vi "Main Game Controller.vi"(8 "error in (no error)":errorcluster, 11 "output cluster":refnum<class "Game.lvclass">) -> (0 "error out":errorcluster)   [LabVIEW 2021, in "Game.lvclass"]
uses:
  Application/Game.lvclass
  GameEl_class/private/Enum Direction.ctl
  Application/Shield.ctl
  Application/Grapes.ctl
  Application/Backgroud_v2.ctl
  <vilib>/Platform/TimedLoop/XDataNode/timing_clust.ctl
  <vilib>/Platform/TimedLoop/XDataNode/nitl_modes.ctl
  <vilib>/Platform/TimedLoop/XDataNode/wakeup.ctl
  Application/Game.lvclass/Game.ctl
  e26eec9f-965e-4c3b-b51e-9e299e1f8818.vi
  49b93924-5950-4f5a-b15f-497dbc55912f.vi
  Application/Globales Snake.vi
  <vilib>/platform/TimedLoop/XDataNode/XDataNode.xnode
  GameEl_class/GameEl.lvclass
  Snake_class/Snake.lvclass
  <vilib>/Platform/TimedLoop/XDataNode/XDNodeRunTimeDep.lvlib
  Board Game_class/Board Game.lvclass
  Imposible_Snake_v2/LVApp/Modules/Sound Manager/Sound Manager.lvlib
panel:
  out "Image Ring":u16(ring)
  out "Star":bool
  in  "Grapes":T1
  in  "Shield":T2
  in  "Studios":bool caption="Creator 2"
  in  "Creator":bool
  out "TIME":string
  out "SCORE":string
  out "Board Game":u32[][](array[colorbox])
  out "Background":T3=1
  in  "Usert Stop Game":bool
  in  "Pause/Resume":bool
  out "Direction":T4
  out "Current Score":u16
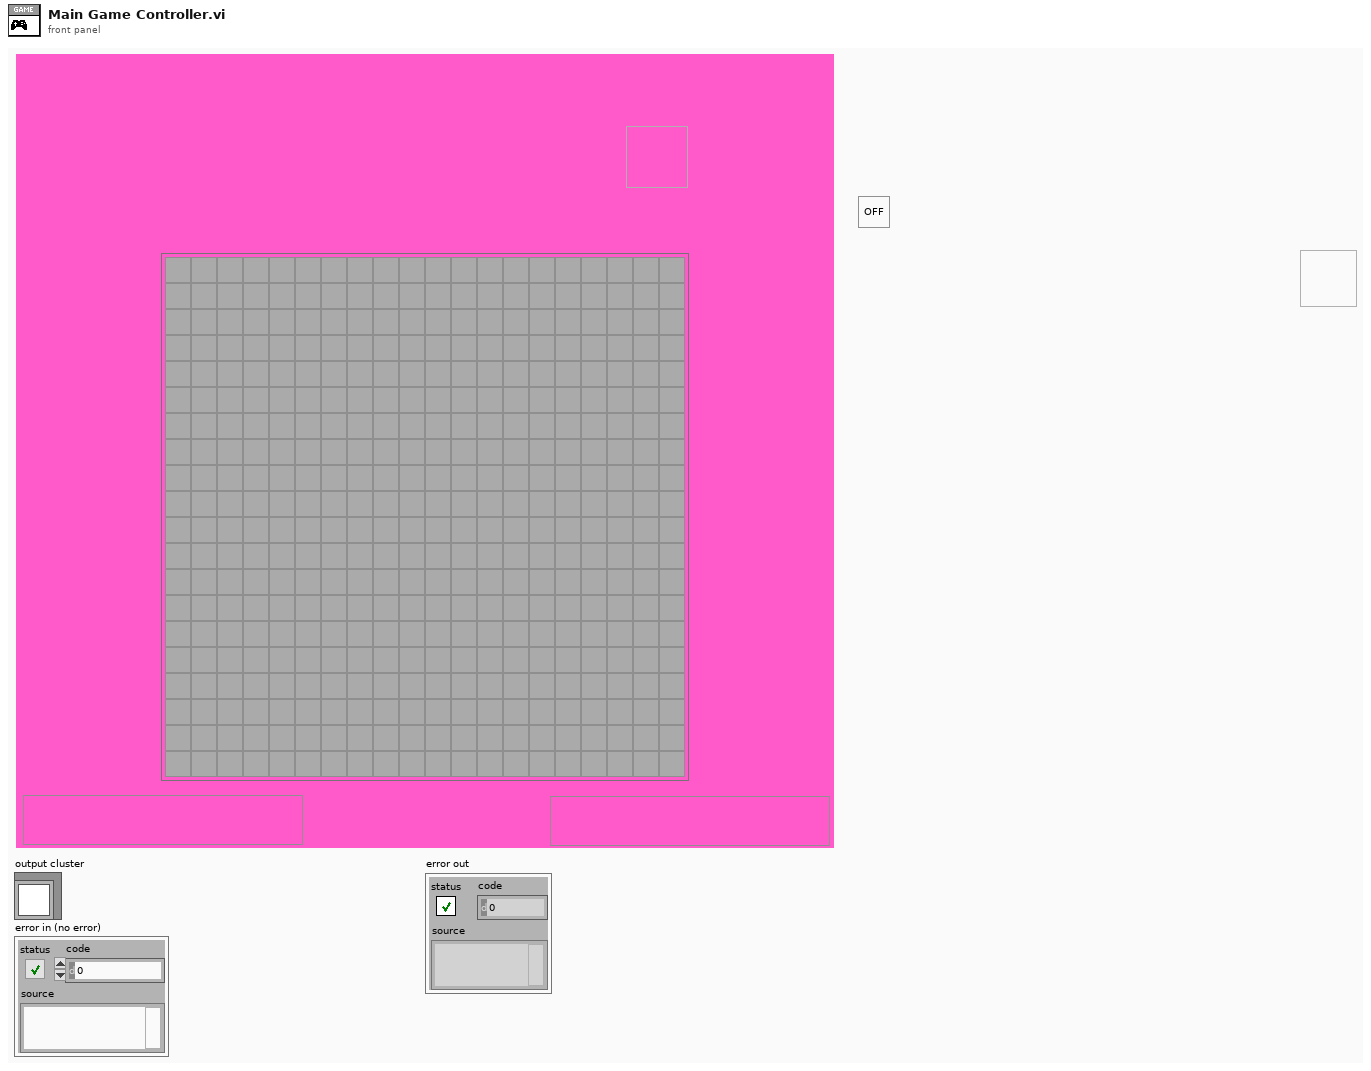
[diagram p1: front panel]
types:
  T1 = typedef "Game.lvclass/Grapes.ctl" = u16
  T2 = typedef "Game.lvclass/Shield.ctl" = u16
  T3 = typedef "Game.lvclass/Backgroud_v2.ctl" = u16
  T4 = typedef "GameEl.lvclass/Enum Direction.ctl" = enum16{"Up", "Down", "Forward", "Backward"}
  T5 = typedef "XDNodeRunTimeDep.lvlib/timing_clust.ctl" = cluster{"Expected End [f-1]":u64, "Actual End [f-1]":u64, "Finished Late? [f-1]":bool, "Expected End [i-1]":u64, "Actual End [i-1]":u64, "Finished Late? [i-1]":bool, "Expected Start [i]":u64, "Actual Start [i]":u64, "Expected Start [f]":u64, "Actual Start [f]":u64, "Source Name":string, "Structure Name":string, "Period":i64, "Deadline":i64, "Offset":i64, "Start":i64, "Priority":i32, "Timeout":i32, "Mode":T6, "Wakeup Reason":T7, "Error":errorcluster, "Source Type":string, "Secondary Source Type":string, "Global End Time":u64, "Global Start Time":u64, "Frame Duration":u64, "Iteration Duration":u64, "Assigned CPU":i32, "I/O Scan Engine Mode":u32}
  T6 = typedef "XDNodeRunTimeDep.lvlib/nitl_modes.ctl" = enum32{"No Change", "Process missed periods, maintain original phase", "Discard missed periods, maintain original phase", "Process missed periods, ignore original phase", "Discard missed periods, ignore original phase"}
  T7 = typedef "XDNodeRunTimeDep.lvlib/wakeup.ctl" = enum32{"Normal", "Aborted", "Asynchronous wakeup", "Timing source error", "Timed loop error", "Timeout"}
  T8 = enum8{"Enabled", "Disabled", "Disabled and Grayed Out"}
  T9 = cluster{"Event Registration Refnum":refnum<event-registration>}
  T10 = enum32{"invalid app kind", "Development System", "Run Time System", "Student Edition", "Embedded LabVIEW", "Evaluation", "Custom"}
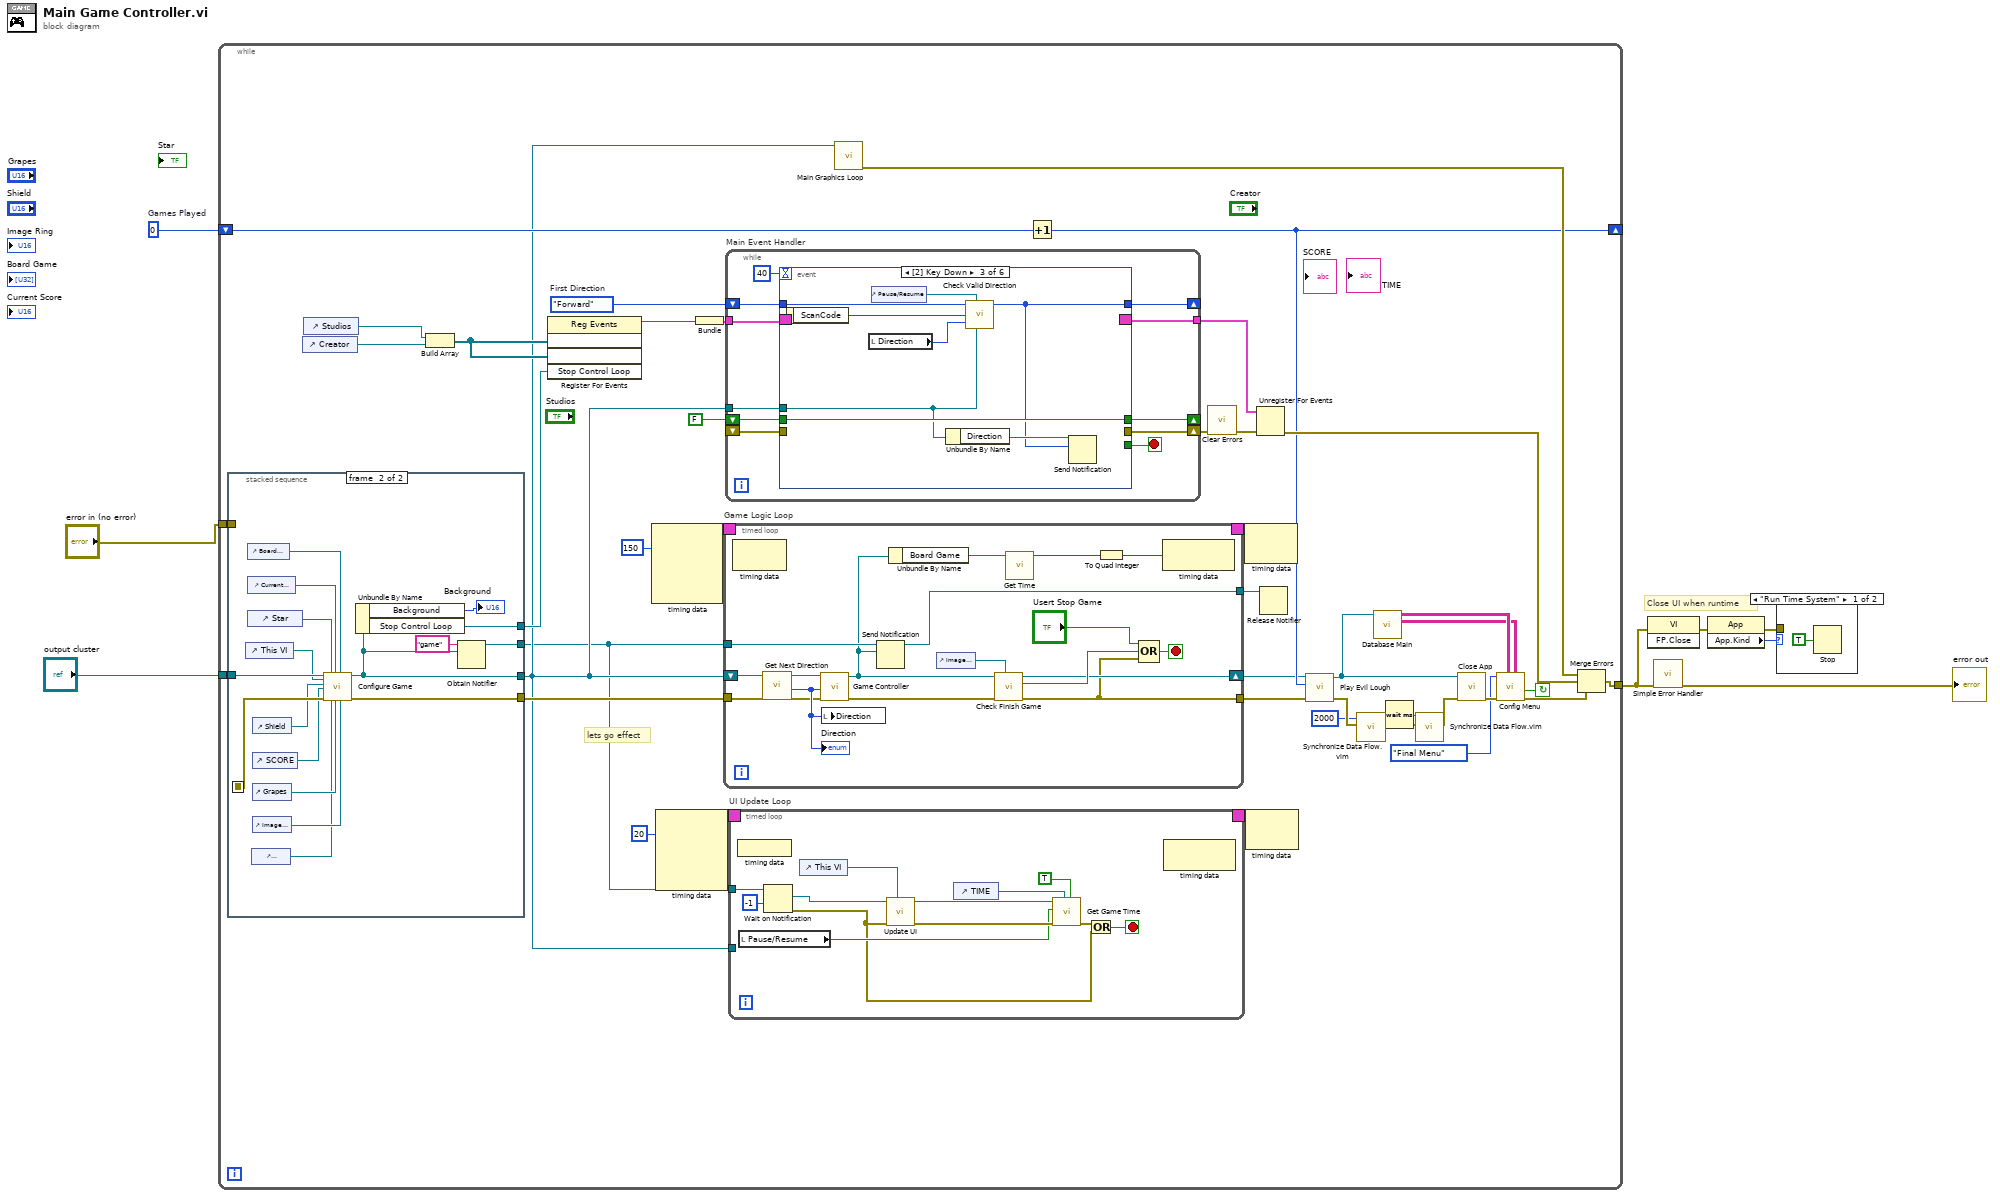
[diagram p0: block diagram]
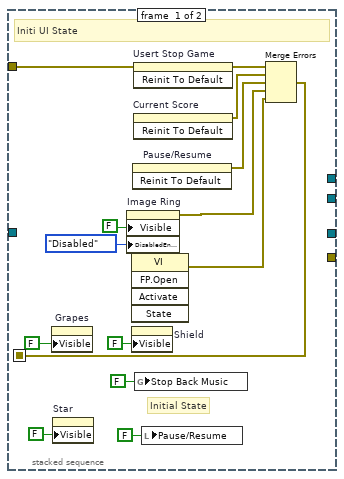
[diagram p2: hidden frame]
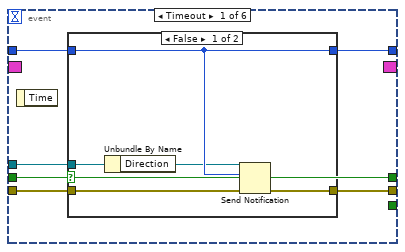
[diagram p3: hidden frame]
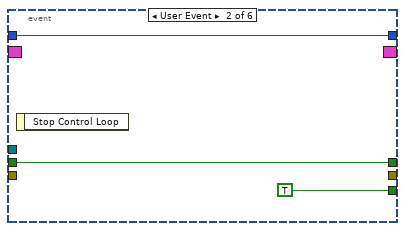
[diagram p5: hidden frame]
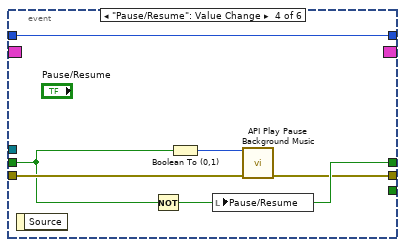
[diagram p6: hidden frame]
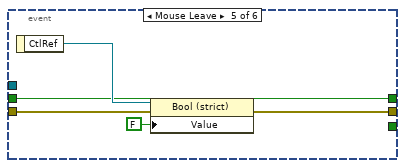
[diagram p7: hidden frame]
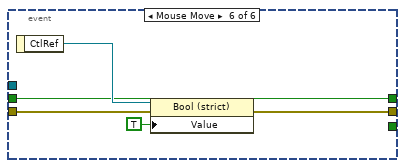
[diagram p8: hidden frame]
diagram:
  w8 = 0  # Games Played
  # "Close UI when runtime"
  n1 = while {
    tunnel: [w43] -> w5
    tunnel: "output cluster" -> [w41]
    shift-right: [w39] -> _
    shift-left: w8 -> [w40]
    tunnel: "error in (no error)" -> [w10]
    stop <- w34 continue-if-true
    w50 = Enum_Direction."Forward"  # First Direction
    # "lets go effect"
    n2 = stacked-sequence {
      seq-local: [w105 _] -> [_ w126]
      tunnel: [_ w125] -> w29
      tunnel: [_ w111] -> w13
      tunnel: [_ w122] -> w44
      tunnel: w41 -> [_ w117]
      tunnel: [_ w110] -> w12
      tunnel: w10 -> [w96 _]
      frame #0 {
        # "Initial State"
        # "Initi UI State"
        n3 = property on="Grapes" class="Ring (strict)"("Visible"=FALSE) -> ()  [unwired: 2 in, 2 out]
        n4 = property on="Star" class="Bool (strict)"("Visible"=FALSE) -> ()  [unwired: 2 in, 2 out]
        n5 = property on="Image Ring" class="Ring (strict)"("Visible"=FALSE, "DisabledEnum"=T8."Disabled" ("Disabled")) -> (error out=w101:errorcluster)  [unwired: 2 in, 1 out]
        n6 = invoke class="VI" method="FP.Open"() -> (error out=w106:errorcluster)  [unwired: 5 in, 4 out]
        n7 = property on="Shield" class="Ring (strict)"("Visible"=FALSE) -> ()  [unwired: 2 in, 2 out]
        n8 = invoke on="Pause/Resume" class="Bool (strict)" method="Reinit To Default"() -> (error out=w107:errorcluster)  [unwired: 3 in, 2 out]
        n9 = invoke on="Usert Stop Game" class="Bool (strict)" method="Reinit To Default"(error in=w96) -> (error out=w109:errorcluster)  [unwired: 2 in, 2 out]
        n10 = invoke on="Current Score" class="DigNum (strict)" method="Reinit To Default"() -> (error out=w108:errorcluster)  [unwired: 3 in, 2 out]
        n11 = global write "Globales Snake.vi" "Stop Back Music"(FALSE ("Stop Back Music")) -> ()
        n12 = local write "Pause/Resume"(FALSE ("Pause/Resume")) -> ()
        n13 = Merge Errors(w109, w108, w107, w101, w106) -> (w105:errorcluster)
      }
      frame #1 {
        n14 = control-ref of="This VI"() -> (w113:refnum<vi>)
        n15 = control-ref of="Board Game"() -> (w124:refnum<vi>)
        n16 = control-ref of="Current Score"() -> (w123:refnum<vi>)
        n17 = control-ref of="Star"() -> (w114:refnum<vi>)
        n18 = control-ref of="Background"() -> (w116:refnum<vi>)
        n19 = control-ref of="Shield"() -> (w121:refnum<vi>)
        n20 = control-ref of="SCORE"() -> (w120:refnum<vi>)
        n21 = control-ref of="Grapes"() -> (w119:refnum<vi>)
        n22 = control-ref of="Image Ring"() -> (w118:refnum<vi>)
        n23 = call "Configure Game.vi"("input cluster"=w117, "This VI"=w113, "Shield"=w121, "SCORE"=w120, "error in (no error)"=w126, "STAR"=w114, "Background"=w116, "Score"=w123, "Grapes"=w119, "Board Game"=w124, "Image Ring"=w118) -> ("Application out"=w111:refnum<class "Game.lvclass">, "error out"=w125:errorcluster)  [unwired: 7 in]
        n24 = Unbundle By Name(w111) -> ("Background"=→"Background":u16, "Stop Control Loop"=w122:refnum<user-event>)
        n25 = Obtain Notifier(name (unnamed)="game", notification data type=w111) -> (notifier out=w110:refnum<notifier>)  [unwired: 2 in, 2 out]
      }
    }
    n26 = control-ref of="Creator"() -> (w28:refnum<vi>)
    n27 = control-ref of="Studios"() -> (w27:refnum<vi>)
    n28 = Build Array(w27, w28) -> (w26:refnum<vi>[])
    n29 = register-events(w26, w26, w44) -> (reference out=w51:refnum<event-registration>)  [unwired: 2 in, 1 out]
    n30 = node-c288(i64 150 ("Period")) -> (w18:T5)  [unwired: 3 in]
    n31 = node-c288(i64 20 ("Period")) -> (w15:T5)  [unwired: 3 in]
    n32 = Bundle("Event Registration Refnum"=w51) -> (w30:T9)  [unwired: 1 in]
    n33 = timed-loop "Game Logic Loop" {
      tunnel: w29 -> [w81]
      tunnel: [w77] -> w37
      shift-right: [w79] -> w38
      shift-left: w13 -> [w86]
      timing: w18 -> [_]
      timing-out: [_] -> w17
      tunnel: w12 -> [w73]
      tunnel: [w70] -> w9
      stop <- w71 stop-if-true
      n34 = node-c288() -> ()  [unwired: 1 in, 1 out]
      n35 = call "Get Next Direction.vi"("error in (no error)"=w81, "Application in"=w86) -> ("error out"=w78:errorcluster, "Direction"=w83:T4, "Application out"=w85:refnum<class "Game.lvclass">)  [unwired: 7 in]
      "Direction" <- w83
      n36 = call "Game Controller.vi"("error in (no error)"=w78, "Direction"=w83, "Application in"=w85) -> ("error out"=w80:errorcluster, "Application out"=w72:refnum<class "Game.lvclass">)  [unwired: 7 in]
      n37 = local write "Direction"(w83) -> ()
      n38 = Send Notification(notification=w72, notifier=w73) -> (notifier out=w70:refnum<notifier>)  [unwired: 1 in, 1 out]
      n39 = Unbundle By Name(w72) -> ("Board Game"=w76:refnum<class "Board Game.lvclass">)
      n40 = control-ref of="Image Ring"() -> (w84:refnum<vi>)
      n41 = call "Check Finish Game.vi"("Game Result"=w84, "error in (no error)"=w80, "Application in"=w72) -> ("error out"=w77:errorcluster, "Finish Game?"=w82:bool, "Application out"=w79:refnum<class "Game.lvclass">)  [unwired: 6 in]
      n42 = call "Get Time.vi"("Board Game in"=w76) -> ("Time"=w75:u32)  [unwired: 9 in, 1 out]
      n43 = To Quad Integer(1:w75) -> (0:w74:i64)
      n44 = Compound Arithmetic op=OR("Usert Stop Game", w82, w77) -> (w71:bool)
      n45 = node-c288(w74) -> ()  [unwired: 1 out]
    }
    n46 = while "Main Event Handler" {
      tunnel: w30 -> [w137]
      tunnel: [w135] -> w46
      shift-right: [w133] -> _
      shift-left: w50 -> [w131]
      tunnel: w13 -> [w132]
      shift-right: [w129] -> w48
      shift-left: _ -> [w130]
      shift-right: [w127] -> _
      shift-left: FALSE -> [w128]
      stop <- w136 stop-if-true
      n47 = event shown="[2] Key Down" {
        selector: w137 -> [_ _ _ _ _ _]
        dyn-events: [_ _ _ _ _ _] -> w135
        timeout: 40 -> [_ _ _ _ _ _]
        tunnel: [_ TRUE _ _ _ _] -> w136
        tunnel: [w139 w152 w154 w167 _ _] -> w133
        tunnel: w132 -> [w143 _ w155 _ _ _]
        tunnel: w131 -> [w140 w152 w160 w167 _ _]
        tunnel: w130 -> [w141 _ _ w164 w172 w177]
        tunnel: [w142 _ _ w165 w171 w176] -> w129
        tunnel: w128 -> [w138 w151 w161 w163 w168 w173]
        tunnel: [w138 w151 w161 w166 w168 w173] -> w127
        event Timeout {
          n48 = event-data() -> ()  [unwired: 1 in, 1 out]
          n49 = case shown="False" w138 {
            tunnel: w143 -> [w148 _]
            tunnel: [w147 w149] -> w142
            tunnel: w141 -> [w146 w149]
            tunnel: w140 -> [w145 w150]
            tunnel: [w145 w150] -> w139
            frame False {
              n50 = Unbundle By Name(w148) -> ("Direction"=w144:refnum<notifier>)
              n51 = Send Notification(notification=w145, notifier=w144, error in (no error)=w146) -> (error out=w147:errorcluster)  [unwired: 1 out]
            }
            frame True {
            }
          }
        }
        event User Event {
          n52 = event-data() -> ()  [unwired: 1 in, 1 out]
        }
        event Key Down {
          n53 = event-data() -> ("ScanCode"=w158:i16)  [unwired: 1 in]
          n54 = local read "Direction"() -> (w159:T4)
          n55 = control-ref of="Pause/Resume"() -> (w157:refnum<vi>)
          n56 = Unbundle By Name(w155) -> ("Direction"=w156:refnum<notifier>)
          n57 = call "Check Valid Direction.vi"("Application out"=w155, "Pause/Resume Ref"=w157, "Last Movement"=w159, "ScanCode"=w158, "Current Direction"=w160) -> ("New Direction"=w154:T4)  [unwired: 6 in]
          n58 = Send Notification(notification=w154, notifier=w156) -> ()  [unwired: 1 in, 2 out]
        }
        event "Pause/Resume": Value Change {
          n59 = event-data() -> ()  [unwired: 1 in, 1 out]
          n60 = Not(x=w163) -> (.not. x?=w166:bool)
          n61 = Boolean To (0,1)(Boolean=w163) -> (0, 1=w162:i16)
          n62 = local write "Pause/Resume"(w166) -> ()
          n63 = call "API Play Pause Background Music.vi"("Error In"=w164, "Function"=w162) -> ("error in (no error)"=w165:errorcluster)  [unwired: 9 in]
        }
        event Mouse Leave {
          n64 = event-data() -> ("CtlRef"=w170:refnum<vi>)  [unwired: 1 in]
          n65 = property class="Bool (strict)"(reference=w170, error in=w172, "Value"=FALSE) -> (error out=w171:errorcluster)  [unwired: 1 out]
        }
        event Mouse Move {
          n66 = event-data() -> ("CtlRef"=w175:refnum<vi>)  [unwired: 1 in]
          n67 = property class="Bool (strict)"(reference=w175, error in=w177, "Value"=TRUE) -> (error out=w176:errorcluster)  [unwired: 1 out]
        }
      }
    }
    n68 = timed-loop "UI Update Loop" {
      timing: w15 -> [_]
      timing-out: [_] -> w14
      tunnel: w12 -> [w62]
      tunnel: w13 -> [_]
      stop <- w60 stop-if-true
      n69 = node-c288() -> ()  [unwired: 1 in]
      n70 = local read "Pause/Resume"() -> (w53:bool)
      n71 = Wait on Notification(notifier=w62, timeout in ms (-1)=-1) -> (notification=w54:refnum<class "Game.lvclass">, error out=w52:errorcluster)  [unwired: 2 in, 2 out]
      n72 = control-ref of="This VI"() -> (w63:refnum<vi>)
      n73 = call "Update UI.vi"("This VI"=w63, "error in (no error)"=w52, "Application in"=w54) -> ("error out"=w57:errorcluster, "Application out"=w55:refnum<class "Game.lvclass">)  [unwired: 7 in]
      n74 = control-ref of="TIME"() -> (w58:refnum<vi>)
      n75 = call "Get Game Time.vi"("update ui"=TRUE, "Time"=w58, "error in (no error)"=w57, "Pause/Resume"=w53, "Application in"=w55) -> ("error out"=w56:errorcluster)  [unwired: 4 in, 2 out]
      n76 = Or(x=w56, y=w52) -> (x .or. y?=w60:bool)
      n77 = node-c288() -> ()  [unwired: 1 in, 1 out]
    }
    n78 = call "Main Graphics Loop.vi"("Application in"=w13) -> ("error out"=w42:errorcluster)  [unwired: 10 in]
    n79 = Increment(x=w40) -> (x+1=w39:i32)
    n80 = call <vilib>:"Clear Errors.vi"("error in (no error)"=w48) -> ("error out"=w47:errorcluster)  [unwired: 5 in, 1 out]
    n81 = node-c288(w17) -> ()  [unwired: 1 out]
    n82 = node-c288(w14) -> ()  [unwired: 1 out]
    n83 = Unregister For Events(event registration refnum=w46, error in=w47) -> (error out=w45:errorcluster)
    n84 = Release Notifier(notifier=w9) -> ()  [unwired: 2 in, 3 out]
    n85 = call "Play Evil Lough.vi"("error in (no error)"=w37, "Number of games"=w39, "Application in"=w38) -> ("error out"=w24:errorcluster, "Application out"=w32:refnum<class "Game.lvclass">)  [unwired: 7 in]
    n86 = call "Synchronize Data Flow.vim"("input 2"=w24, "input 1"=u32 2000 ("milliseconds to wait")) -> ("output 2"=w21:errorcluster, "output 1"=w22:u32)  [unwired: 2 in, 2 out]
    n87 = call "Database Main.vi"("Application.lvclass"=w32) -> ("Stats"=w25:string[][], "Games"=w31:string[][])  [unwired: 9 in]
    n88 = Wait (ms)(milliseconds to wait=w22) -> (millisecond timer value=w20:u32)
    n89 = call "Synchronize Data Flow.vim"("input 2"=w21, "input 1"=w20) -> ("output 2"=w19:errorcluster)  [unwired: 2 in, 3 out]
    n90 = call "Close App.vi"("error in (no error)"=w19, "Application in"=w32) -> ("error out"=w36:errorcluster)  [unwired: 9 in]
    n91 = call "Config Menu.vi"("Stats"=w25, "Data Out"=w31, "error in (no error)"=w36, "Enum"=enum16{"Initial Menu", "Final Menu"}."Final Menu") -> ("error out"=w33:errorcluster, "Play/stop"=w34:bool)  [unwired: 5 in, 1 out]
    n92 = Merge Errors(w42, w45, w33) -> (w43:errorcluster)
  }
  n93 = invoke class="VI" method="FP.Close"(error in=w5) -> (error out=w4:errorcluster)  [unwired: 2 in, 2 out]
  n94 = call <vilib>:"Simple Error Handler.vi"("error in (no error)"=w5) -> ("error out"=→"error out":errorcluster)  [unwired: 4 in, 4 out]
  n95 = property class="App"(error in=w4) -> (error out=w6:errorcluster, "App.Kind"=w7:T10)  [unwired: 1 in, 1 out]
  n96 = case shown="\"Run Time System\"" w7 {
    tunnel: w6 -> [_ _]
    frame "Run Time System" {
      n97 = Stop(stop? (T)=TRUE) -> ()
    }
    frame Default {
    }
  }
